vi "hmi_simulacionEuler.vi"() -> ()   [LabVIEW 2017]
uses:
  Control 6.ctl
  <vilib>/Platform/TimedLoop/XDataNode/timing_clust.ctl
  <vilib>/Platform/TimedLoop/XDataNode/nitl_modes.ctl
  <vilib>/Platform/TimedLoop/XDataNode/wakeup.ctl
  <vilib>/platform/TimedLoop/XDataNode/XDataNode.xnode
  <vilib>/Platform/TimedLoop/XDataNode/XDNodeRunTimeDep.lvlib
panel:
  in  "Tab Control":enum32{"HMI", "Monitorizacion de flujo"}(tab)
  in  "Presion de salida":dbl caption="MPa"
  in  "Presion de entrada":dbl caption="MPa"
  out "PT-002":dbl caption="MPa"
  out "PT-001":dbl caption="MPa"
  in  "Flujo de entrada":dbl caption="L/min"
  in  "Flujo de salida":dbl caption="L/min"
  out "Boolean 2":bool
  out "FUGA 1":bool
  out "FUGA 2":bool
  out "Boolean":bool
  in  "stop 2":bool
  in  "BOMBA ON/OFF":bool
  out "FT1":bool(c317)
  out "TANQUE\n FLUIDO:AGUA":dbl(slide) scale=0.0..100.0
  in  "valvula 1":bool
  in  "valvula 2":bool
  in  "ts":dbl caption="ms"
  out "TEE 02":bool
  out "TUBERIA 1IN TRAMO 02":bool(c317)
  out "TEE1":bool
  out "Multi-Segment Pipe 2":T1
  out "Multi-Segment Pipe 3":bool(c317)
  out "BOMBA  PERIFERICA1/2 HP":bool
  out "codo90":bool
  out "Multi-Segment Pipe 4":bool(c317)
  out "FT2":bool(c317)
  in  "u1":dbl
  in  "u2":dbl
  in  "tiempo de simulacion":i8=8
  out "FT -001":dbl caption="L/min"
  out "FT-002":dbl caption="L/min"
  out "SENSOR FLUJO 4":bool
  out "SENSOR FLUJO 5":bool
  out "Tiempo":dbl caption="s"
  out "XY Graph":cluster{dbl[], dbl[]}(graph)
  in  "Guardar  a Excel":bool
  in  "Rango de grafica":i16(knob) scale=0.0..100.0
  out "Flujo de entrada y salida":cluster{dbl[], dbl[]}[](graph)
  in  "stop":bool
  # "PVC  1\" FLUJO: AGUA"
  # "PVC  1/2\" FLUJO: AGUA"
  # "FUGA 1"
  # "2.5 m"
  # "PVC  1/2\" FLUJO: AGUA"
  # "FUGA 2"
  # "PVC  1\" FLUJO: AGUA"
  # "9 m"
  # "Grafica de flujo en sensores YF-S201"
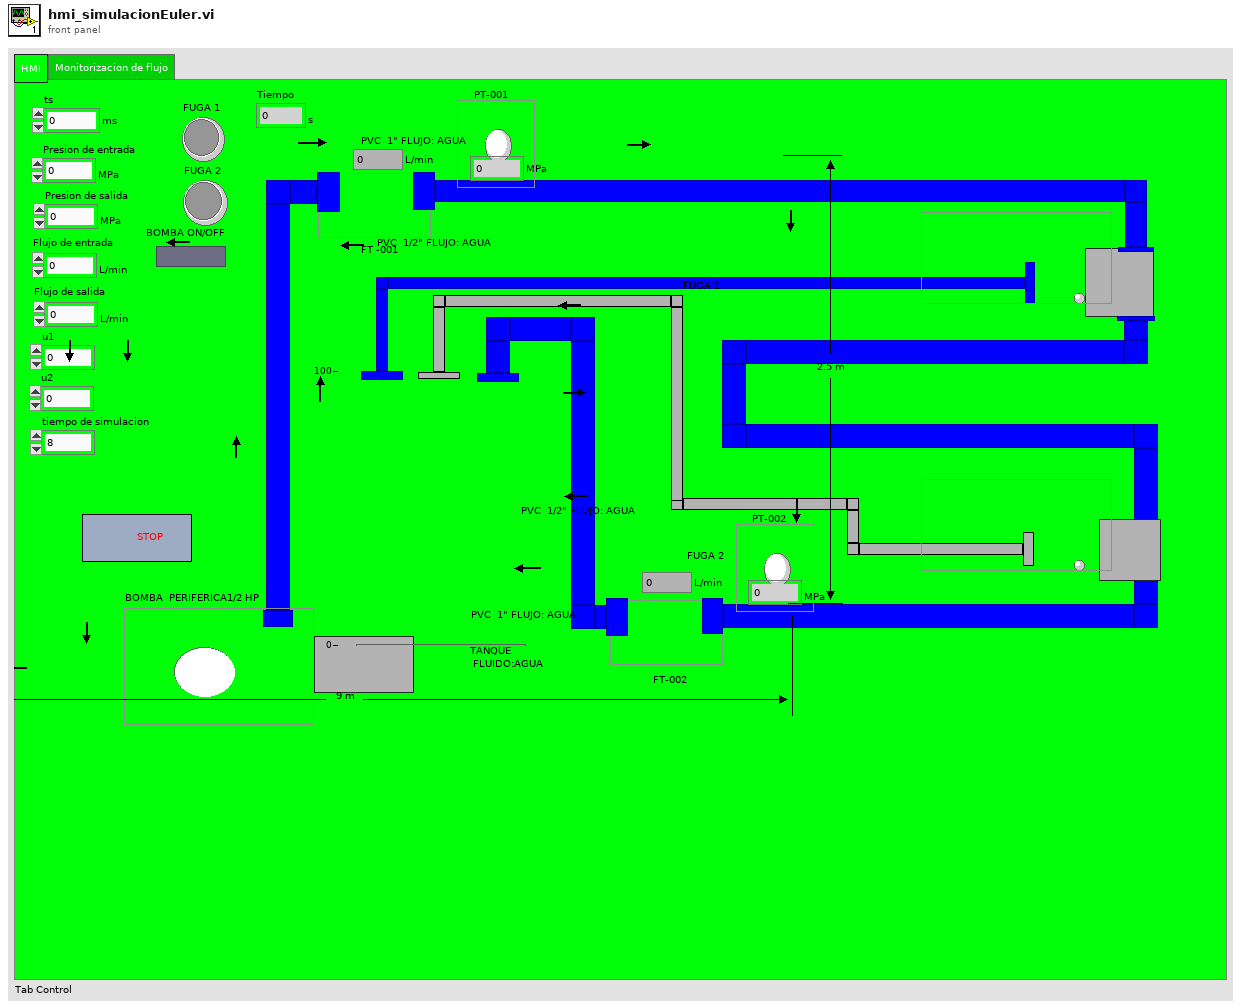
[diagram p1: front panel]
types:
  T1 = typedef "Control 6.ctl" = bool
  T2 = typedef "XDNodeRunTimeDep.lvlib/timing_clust.ctl" = cluster{"Expected End [f-1]":u64, "Actual End [f-1]":u64, "Finished Late? [f-1]":bool, "Expected End [i-1]":u64, "Actual End [i-1]":u64, "Finished Late? [i-1]":bool, "Expected Start [i]":u64, "Actual Start [i]":u64, "Expected Start [f]":u64, "Actual Start [f]":u64, "Source Name":string, "Structure Name":string, "Period":i64, "Deadline":i64, "Offset":i64, "Start":i64, "Priority":i32, "Timeout":i32, "Mode":T3, "Wakeup Reason":T4, "Error":errorcluster, "Source Type":string, "Secondary Source Type":string, "Global End Time":u64, "Global Start Time":u64, "Frame Duration":u64, "Iteration Duration":u64, "Assigned CPU":i32, "I/O Scan Engine Mode":u32}
  T3 = typedef "XDNodeRunTimeDep.lvlib/nitl_modes.ctl" = enum32{"No Change", "Process missed periods, maintain original phase", "Discard missed periods, maintain original phase", "Process missed periods, ignore original phase", "Discard missed periods, ignore original phase"}
  T4 = typedef "XDNodeRunTimeDep.lvlib/wakeup.ctl" = enum32{"Normal", "Aborted", "Asynchronous wakeup", "Timing source error", "Timed loop error", "Timeout"}
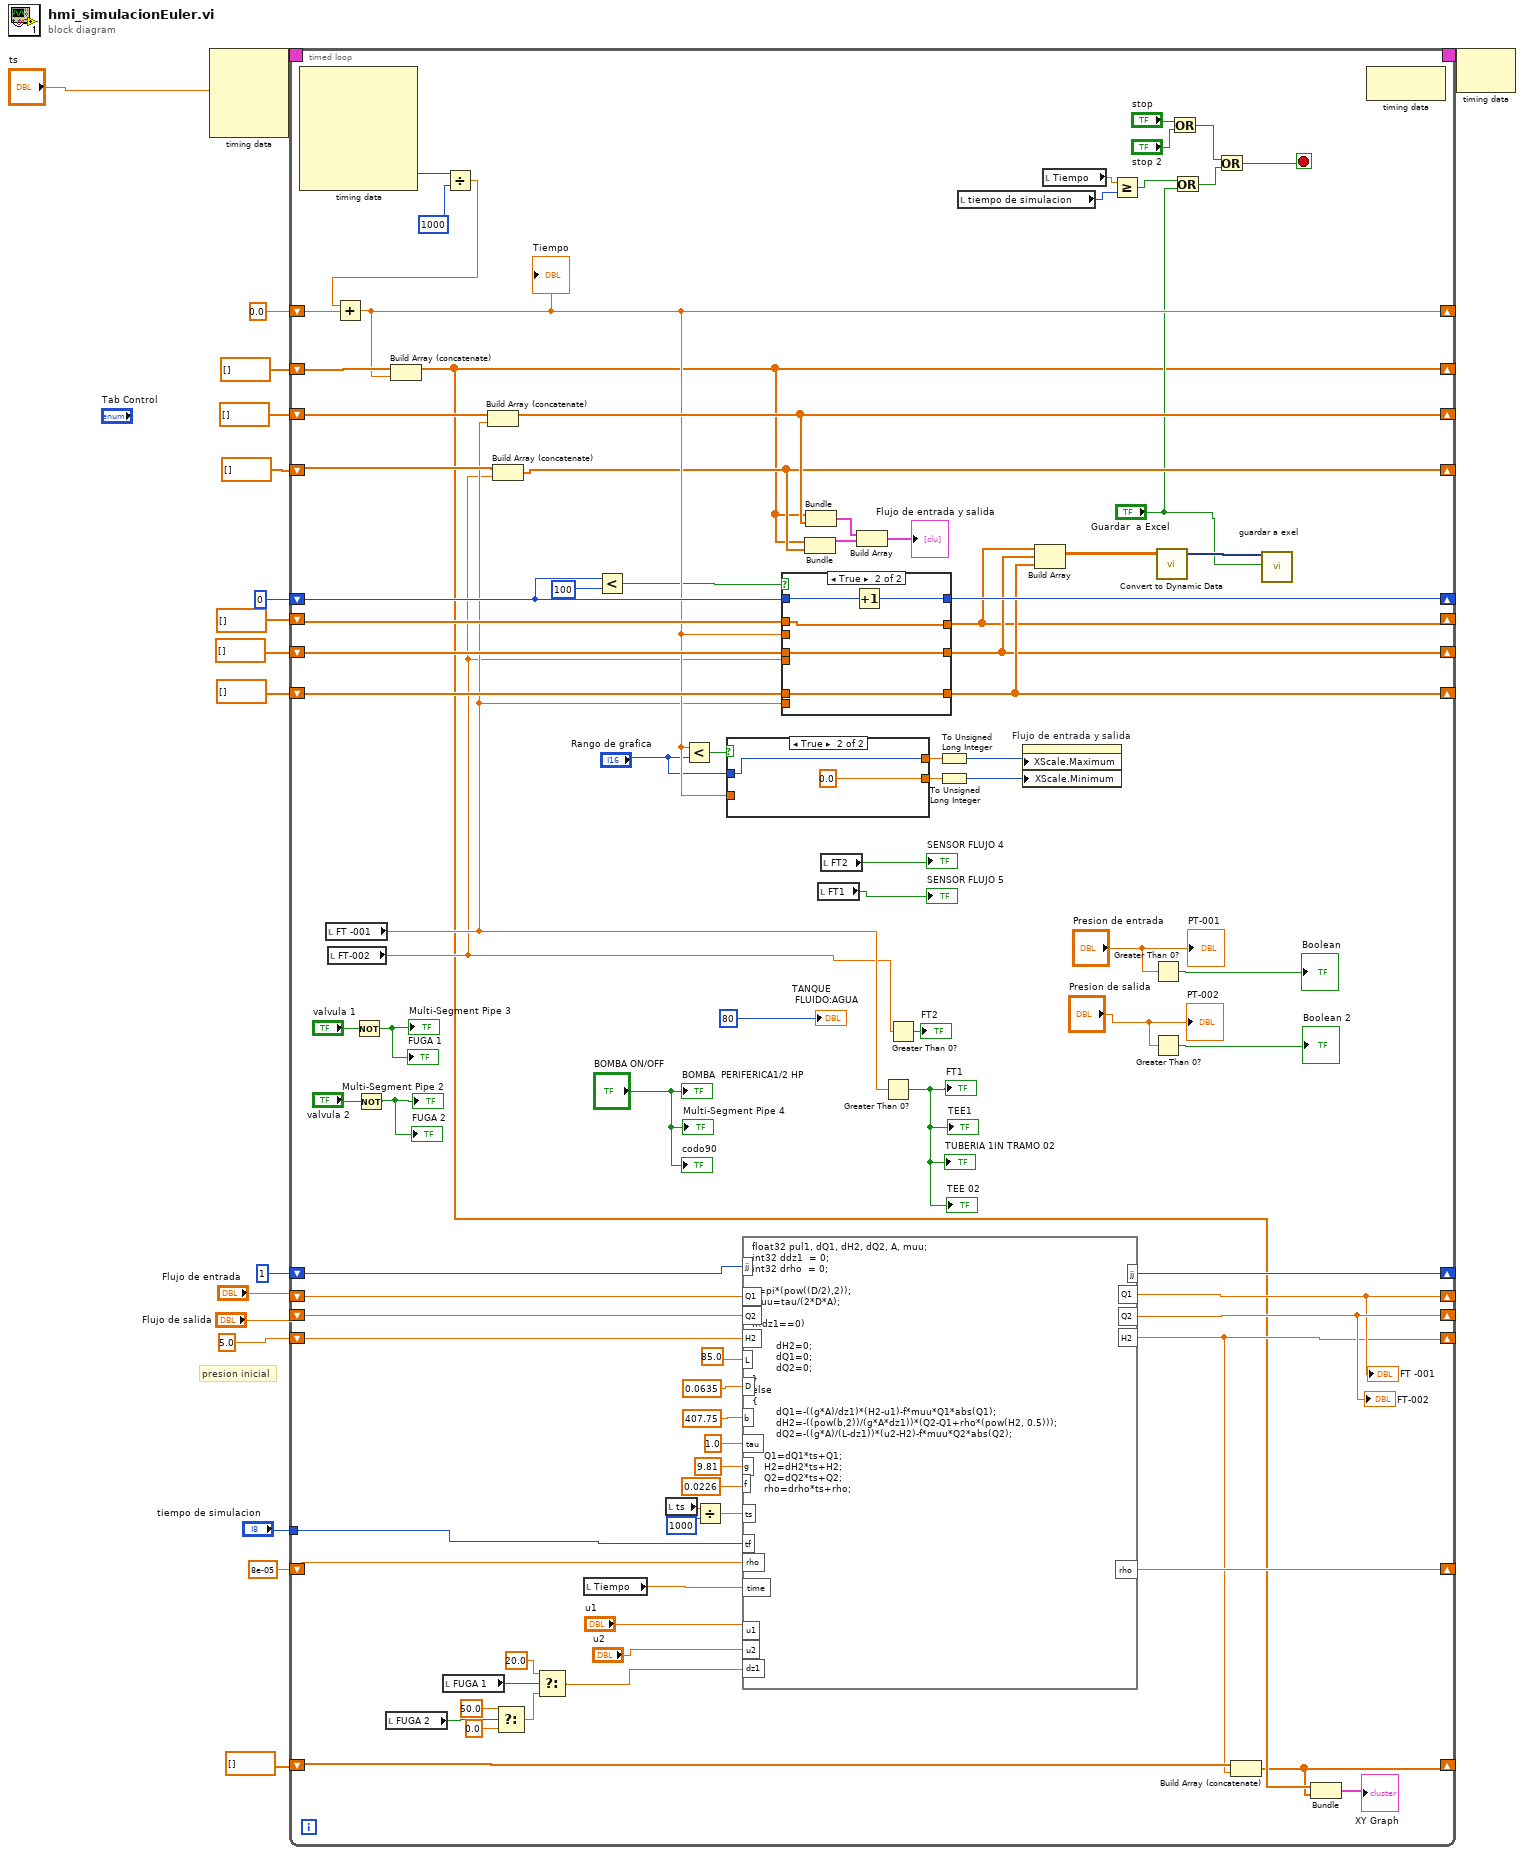
[diagram p0: block diagram]
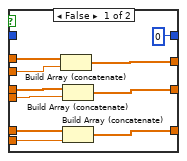
[diagram p2: hidden frame]
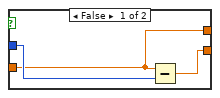
[diagram p3: hidden frame]
diagram:
  # "presion inicial"
  n1 = node-c288("ts") -> (w10:T2)  [unwired: 3 in]
  n2 = timed-loop {
    shift-right: [w20] -> _
    shift-left: dbl[] [] -> [w107]
    shift-right: [w90] -> _
    shift-left: 0.0 -> [w108]
    shift-right: [w100] -> _
    shift-left: dbl[] [] -> [w105]
    shift-right: [w80] -> _
    shift-left: dbl[] [] -> [w106]
    shift-right: [w96] -> _
    shift-left: 0 -> [w97]
    shift-right: [w91] -> _
    shift-left: dbl[] [] -> [w94]
    shift-right: [w92] -> _
    shift-left: dbl[] [] -> [w93]
    shift-right: [w89] -> _
    shift-left: dbl[] [] -> [w95]
    timing: w10 -> [_]
    timing-out: [_] -> w9
    shift-right: [w38] -> _
    shift-left: "Flujo de salida" -> [w40]
    shift-right: [w37] -> _
    shift-left: "Flujo de entrada" -> [w39]
    shift-right: [w33] -> _
    shift-left: 5.0 -> [w54]
    shift-right: [w48] -> _
    shift-left: i64 1 -> [w51]
    shift-right: [w49] -> _
    shift-left: 8e-05 ("input variable") -> [w50]
    tunnel: "tiempo de simulacion" -> [w43]
    shift-right: [w19] -> _
    shift-left: dbl[] [] -> [w34]
    stop <- w99 stop-if-true
    n3 = node-c288() -> (w66:i64)  [unwired: 1 in, 6 out]
    n4 = local read "FT -001"() -> (w36:dbl)
    n5 = local read "FT-002"() -> (w35:dbl)
    n6 = Not(x="valvula 1") -> (.not. x?=→"Multi-Segment Pipe 3" →"FUGA 1":bool)
    n7 = Not(x="valvula 2") -> (.not. x?=→"Multi-Segment Pipe 2" →"FUGA 2":bool)
    n8 = local read "FUGA 2"() -> (w29:bool)
    n9 = local read "FUGA 1"() -> (w31:bool)
    n10 = Divide(x=w66, y=i64 1000) -> (x/y=w65:dbl)
    n11 = Add(x=w65, y=w108) -> (x+y=w90:dbl)
    "Tiempo" <- w90
    n12 = Build Array (concatenate)(w107, w90) -> (w20:dbl[])
    n13 = Build Array (concatenate)(w105, w36) -> (w100:dbl[])
    n14 = Build Array (concatenate)(w106, w35) -> (w80:dbl[])
    n15 = Select(t=50.0, s=w29, f=0.0) -> (s? t:f=w28:dbl)
    n16 = Select(t=20.0, s=w31, f=w28) -> (s? t:f=w32:dbl)
    n17 = local read "Tiempo"() -> (w41:dbl)
    n18 = Less?(x=w97, y=u32 100) -> (x < y?=w81:bool)
    n19 = local read "ts"() -> (w56:dbl)
    n20 = Less?(x=w90, y="Rango de grafica") -> (x < y?=w102:bool)
    n21 = Divide(x=w56, y=1000) -> (x/y=w55:dbl)
    n22 = case shown="True" w102 {
      tunnel: "Rango de grafica" -> [w128 w130]
      tunnel: [w127 w130] -> w86
      tunnel: [w129 0.0] -> w84
      tunnel: w90 -> [w127 _]
      frame False {
        n23 = Subtract(x=w127, y=w128) -> (x-y=w129:dbl)
      }
      frame True {
      }
    }
    n24 = formula code="float32 pul1, dQ1, dH2, dQ2, A, muu;\nint32 ddz1  = 0;\nint32 drho  = 0;\n\nA=pi*(pow((D/2),2));\nmuu=tau/(2*D*A);\n\nif(dz1==0)\n{\n        dH2=0;\n        dQ1=0;\n        dQ2=0;\n}\nelse \n{\n        dQ1=-((g*A)/dz1)*(H2-u1)-f*muu*Q1*abs(Q1);\n        dH2=-((pow(b,2))/(g*A*dz1))*(Q2-Q1+rho*(pow(H2, 0.5)));\n        dQ2=-((g*A)/(L-dz1))*(u2-H2)-f*muu*Q2*abs(Q2);\n}\n    Q1=dQ1*ts+Q1;\n    H2=dH2*ts+H2;    \n    Q2=dQ2*ts+Q2;\n    rho=drho*ts+rho;"("L"=85.0, "D"=0.0635, "b"=407.75 ("input variable"), "tau"=1.0 ("input variable"), "g"=9.81 ("input variable"), "Q1"=w39, "Q2"=w40, "f"=0.0226 ("input variable"), "ts"=w55, "tf"=w43, "rho"=w50, "H2"=w54, "time"=w41, "u1"="u1", "u2"="u2", "dz1"=w32, "jj"=w51) -> ("rho"=w49:dbl, "Q1"=w37:dbl, "Q2"=w38:dbl, "H2"=w33:dbl, "jj"=w48:i64)
    "FT -001" <- w37
    "FT-002" <- w38
    n25 = case shown="True" w81 {
      tunnel: w97 -> [_ w126]
      tunnel: [u32 0 w125] -> w96
      tunnel: w95 -> [w120 w122]
      tunnel: w35 -> [w118 _]
      tunnel: [w121 w124] -> w91
      tunnel: w94 -> [w119 w124]
      tunnel: w36 -> [w116 _]
      tunnel: w93 -> [w117 w123]
      tunnel: [w115 w123] -> w92
      tunnel: [w114 w122] -> w89
      tunnel: w90 -> [w113 _]
      frame False {
        n26 = Build Array (concatenate)(w120, w113) -> (w114:dbl[])
        n27 = Build Array (concatenate)(w119, w118) -> (w121:dbl[])
        n28 = Build Array (concatenate)(w117, w116) -> (w115:dbl[])
      }
      frame True {
        n29 = Increment(x=w126) -> (x+1=w125:u32)
      }
    }
    n30 = Bundle(w20, w80) -> (w103:cluster{dbl[], dbl[]})  [unwired: 1 in]
    n31 = Bundle(w20, w100) -> (w104:cluster{dbl[], dbl[]})  [unwired: 1 in]
    n32 = local read "FT1"() -> (→"SENSOR FLUJO 5":bool)
    n33 = local read "FT2"() -> (→"SENSOR FLUJO 4":bool)
    n34 = Build Array(w104, w103) -> (→"Flujo de entrada y salida":cluster{dbl[], dbl[]}[])
    n35 = Greater Than 0?(x=w36) -> (x > 0?=→"TUBERIA 1IN TRAMO 02" →"TEE1" →"TEE 02" →"FT1":bool)
    n36 = Greater Than 0?(x=w35) -> (x > 0?=→"FT2":bool)
    n37 = To Unsigned Long Integer(number=w86) -> (unsigned 32bit integer=w85:u32)
    n38 = To Unsigned Long Integer(number=w84) -> (unsigned 32bit integer=w83:u32)
    n39 = local read "tiempo de simulacion"() -> (w42:i8)
    n40 = property on="Flujo de entrada y salida" class="XYGraph (strict)"("XScale.Maximum"=w85, "XScale.Minimum"=w83) -> ()  [unwired: 2 in, 2 out]
    n41 = Build Array(w89, w91, w92) -> (w87:dbl[][])
    n42 = local read "Tiempo"() -> (w45:dbl)
    n43 = Greater Or Equal?(x=w45, y=w42) -> (x >= y?=w44:bool)
    n44 = Greater Than 0?(x="Presion de entrada") -> (x > 0?=→"Boolean":bool)
    n45 = Greater Than 0?(x="Presion de salida") -> (x > 0?=→"Boolean 2":bool)
    n46 = call "Convert to Dynamic Data"("2D Array"=w87) -> ("Dynamic Data Type"=w88:dynamicdata)  [unwired: 3 in]
    n47 = Or(x="stop", y="stop 2") -> (x .or. y?=w74:bool)
    n48 = Or(x=w44, y="Guardar  a Excel") -> (x .or. y?=w46:bool)
    n49 = Or(x=w74, y=w46) -> (x .or. y?=w99:bool)
    n50 = Build Array (concatenate)(w34, w33) -> (w19:dbl[])
    n51 = call "guardar a exel"("Signals"=w88, "Enable"="Guardar  a Excel") -> ()  [unwired: 15 in, 3 out]
    n52 = Bundle(w20, w19) -> (→"XY Graph":cluster{dbl[], dbl[]})  [unwired: 1 in]
    n53 = node-c288() -> ()  [unwired: 1 in, 1 out]
    "TANQUE\n FLUIDO:AGUA" <- 80
    "BOMBA  PERIFERICA1/2 HP" <- "BOMBA ON/OFF"
    "codo90" <- "BOMBA ON/OFF"
    "Multi-Segment Pipe 4" <- "BOMBA ON/OFF"
    "PT-001" <- "Presion de entrada"
    "PT-002" <- "Presion de salida"
  }
  n54 = node-c288(w9) -> ()  [unwired: 1 out]
